vi "Write TOML File.vi"   [LabVIEW 2019, in "BlueTOMLSerializer.lvlib"]
uses:
  BlueTOMLSerializer.lvlib
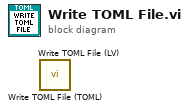
[diagram p0: block diagram]
diagram:
  n1 = call "Write TOML File (TOML).vi"() -> ()  [unwired: 11 in, 1 out]
  n2 = call "Write TOML File (LV).vi"() -> ()  [unwired: 11 in, 1 out]
